vi "dfd_Multirate Filter Order Estimation.vi"(4 "order option":enum16{"MinNum", "MinEven", "MinOdd"}(ring)=enum."MinEven", 5 "method":u16(ring) items=["Kaiser Window", "Dolph-Chebyshev Window", "Equi-Ripple", "Positive Equi-Ripple"], 6 "band option":enum16{"Normal", "Nyquist", "Alias free"}(ring)=enum."Nyquist", 7 "multirate factor":i32=4, 8 "error in (no error)":errorcluster, 9 "A Stop [dB]":dbl format="%.2f", 10 "roll off":dbl format="%.2f") -> (0 "error out":errorcluster, 2 "dup roll off":dbl format="%.2f", 3 "new order":i32)   [LabVIEW 2017, in "NI_DigFilterLicensed.lvlib"]
uses:
  <vilib>/addons/Digital Filter Design/NI_DigFilterLicensed.lvlib
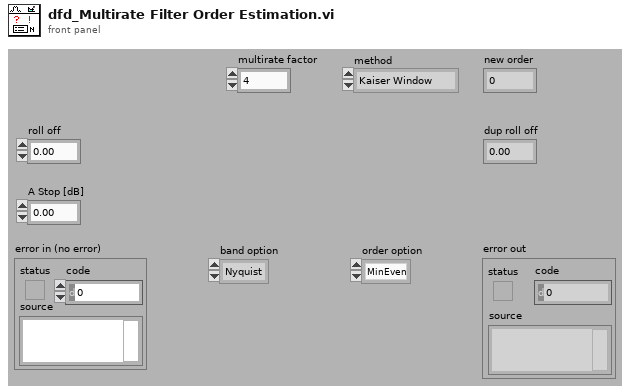
[diagram p1: front panel]
types:
  T1 = enum16{"Lowpass", "Highpass", "Bandpass", "Bandstop"}
  T2 = cluster{"linear value":dbl, "linear value":dbl, bool}
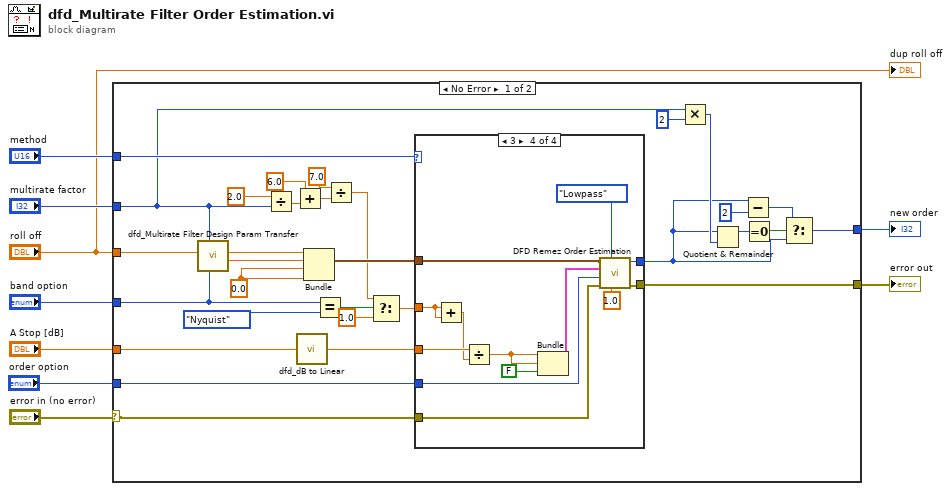
[diagram p0: block diagram]
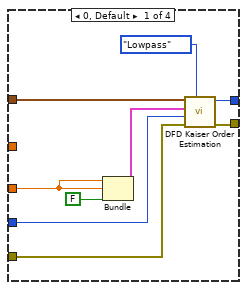
[diagram p2: hidden frame]
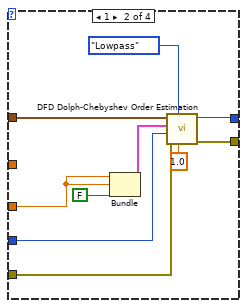
[diagram p3: hidden frame]
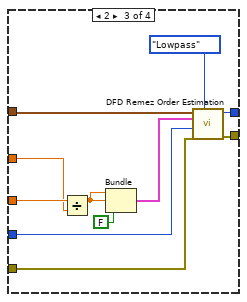
[diagram p4: hidden frame]
diagram:
  n1 = case shown="No Error" "error in (no error)" {
    selector: "error in (no error)" -> [w36 w84]
    tunnel: "roll off" -> [w27 _]
    tunnel: [w40 w84] -> w9
    tunnel: "method" -> [w37 _]
    tunnel: [w29 _] -> w7
    tunnel: "A Stop [dB]" -> [w24 _]
    tunnel: "multirate factor" -> [w11 _]
    tunnel: "band option" -> [w22 _]
    tunnel: "order option" -> [w10 _]
    frame No Error {
      w39 = 0.0
      n2 = call <vilib>:"dfd_Multirate Filter Design Param Transfer.vi"("option"=w22, "multirate factor"=w11, "roll off"=w27) -> ("fstop"=w25:dbl, "fpass"=w26:dbl)  [unwired: 3 in, 4 out]
      n3 = Divide(x=2.0, y=w11) -> (x/y=w16:dbl)
      n4 = Add(x=6.0, y=w16) -> (x+y=w13:dbl)
      n5 = call <vilib>:"dfd_dB to Linear.vi"("dB value"=w24) -> ("linear value"=w23:dbl)  [unwired: 1 in]
      n6 = Bundle("fpass"=w26, "fstop"=w25, w39, w39) -> (w38:cluster{"fpass":dbl, "fstop":dbl, dbl, dbl})  [unwired: 1 out]
      n7 = Equal?(x=w22, y=enum16{"Normal", "Nyquist", "Alias free"}."Nyquist") -> (x = y?=w20:bool)
      n8 = Divide(x=7.0 ("y"), y=w13) -> (x/y=w12:dbl)
      n9 = Select(t=w12, s=w20, f=1.0) -> (s? t:f=w18:dbl)
      n10 = case shown="3" w37 {
        tunnel: w36 -> [w48 w59 w68 w77]
        tunnel: [w47 w58 w66 w79] -> w40
        tunnel: w38 -> [w49 w56 w69 w75]
        tunnel: [w46 w55 w70 w81] -> w30
        tunnel: w23 -> [w44 w53 w62 w74]
        tunnel: w18 -> [_ _ w61 w73]
        tunnel: w10 -> [w41 w50 w60 w71]
        frame 0, Default {
          n11 = Bundle("linear value"=w44, "linear value"=w44, FALSE) -> (w42:T2)  [unwired: 1 out]
          n12 = call <vilib>:"DFD Kaiser Order Estimation.vi"("filter type"=T1."Lowpass", "error in (no error)"=w48, "order option"=w41, "ripple specs"=w42, "freq specs [Hz]"=w49) -> ("error out"=w47:errorcluster, "estimated order"=w46:i32)  [unwired: 1 in, 4 out]
        }
        frame 1 {
          n13 = Bundle("linear value"=w53, "linear value"=w53, FALSE) -> (w51:T2)  [unwired: 1 out]
          n14 = call <vilib>:"DFD Dolph-Chebyshev Order Estimation.vi"("fs [Hz]"=1.0, "filter type"=T1."Lowpass", "error in (no error)"=w59, "order option"=w50, "ripple specs"=w51, "freq specs [Hz]"=w56) -> ("error out"=w58:errorcluster, "estimated order"=w55:i32)  [unwired: 4 out]
        }
        frame 2 {
          n15 = Divide(x=w62, y=w61) -> (x/y=w63:dbl)
          n16 = Bundle(w63, w63, FALSE) -> (w64:cluster{dbl, dbl, bool})  [unwired: 1 out]
          n17 = call <vilib>:"DFD Remez Order Estimation.vi"("filter type"=T1."Lowpass", "error in (no error)"=w68, "order option"=w60, "ripple specs"=w64, "freq specs [Hz]"=w69) -> ("error out"=w66:errorcluster, "estimated order"=w70:i32)  [unwired: 1 in, 4 out]
        }
        frame 3 {
          n18 = Add(x=w73, y=w73) -> (x+y=w72:dbl)
          n19 = Divide(x=w74, y=w72) -> (x/y=w76:dbl)
          n20 = Bundle(w76, w76, FALSE) -> (w80:cluster{dbl, dbl, bool})  [unwired: 1 out]
          n21 = call <vilib>:"DFD Remez Order Estimation.vi"("fs [Hz]"=1.0, "filter type"=T1."Lowpass", "error in (no error)"=w77, "order option"=w71, "ripple specs"=w80, "freq specs [Hz]"=w75) -> ("error out"=w79:errorcluster, "estimated order"=w81:i32)  [unwired: 4 out]
        }
      }
      n22 = Multiply(x=w11, y=2) -> (x*y=w34:i32)
      n23 = Quotient & Remainder(x=w30, y=w34) -> (x-y*floor(x/y)=w33:i32)  [unwired: 1 out]
      n24 = Subtract(x=w30, y=2) -> (x-y=w31:i32)
      n25 = Equal To 0?(x=w33) -> (x = 0?=w28:bool)
      n26 = Select(t=w31, s=w28, f=w30) -> (s? t:f=w29:i32)
    }
    frame Error {
    }
  }
  "new order" <- w7
  "error out" <- w9
  "dup roll off" <- "roll off"
